vi "Control FM sweep.vi"() -> ()   [LabVIEW 2009]
doc: "A wrapper around <B>Set FM sweep.vi</B> that allows you to use either start/stop or center/span frequency controls to set up an FM sweep."
uses:
  FG FM sweep center span control.ctl
  FG FM sweep start stop control.ctl
  Magnet/Oxford/PSSUBS.LLB/PSIO.ctl
  Magnet/Oxford/BUSGEN.LLB/OxfordAddress.ctl
  Tektronix AFG 3000 Series/controls.llb/Voltage.ctl
  Tektronix AFG 3000 Series/Tektronix AFG 3000 Series.lvlib
panel:
  out "Max Delta F":dbl[unit] format="%.3g"
  in  "Overall rep rate":dbl[unit]=50.0 min=0.0 step=0.01 format="%.3g"
  in  "# frequencies":u32=3 min=1 step=1
  in  "center/span":T1 {"span" min=0.0 step=10000.0 format="%.4g"; "center" min=0.0 step=10000.0 format="%.4g"}
  in  "track B field":bool
  in  "RF on/off (ch. 1)":bool
  in  "peak-to-peak voltage":dbl[unit]=1.0 format="%.2g"
  in  "set":bool
  in  "exit":bool
  in  "start/stop":T2 {"stop" min=0.0 step=10000.0 format="%.4g"; "start" min=0.0 step=10000.0 format="%.4g"}
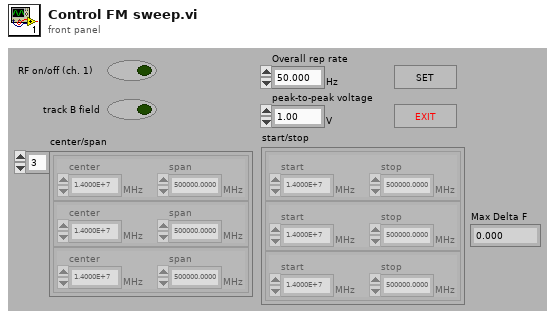
[diagram p1: front panel]
types:
  T1 = typedef "FG FM sweep center span control.ctl" = cluster{"center":dbl[unit], "span":dbl[unit]}[]
  T2 = typedef "FG FM sweep start stop control.ctl" = cluster{"start":dbl[unit], "stop":dbl[unit]}[]
  T3 = typedef "PSIO.ctl" = cluster{"Address":T4, "Version":enum16{"PS", "IPS"}}
  T4 = typedef "OxfordAddress.ctl" = cluster{"Com Port":i32, "ISOBUS Address":i32, "GPIB Address":i16, "Communication":enum16{"RS232", "ISOBUS", "GPIB", "Gateway"}}
  T5 = typedef "Voltage.ctl" = enum16{"amplitude", "offset", "high", "low", "high limit", "low limit"}
  T6 = typedef "LVRectTypeDef.ctl" = cluster{"left":i16, "top":i16, "right":i16, "bottom":i16}
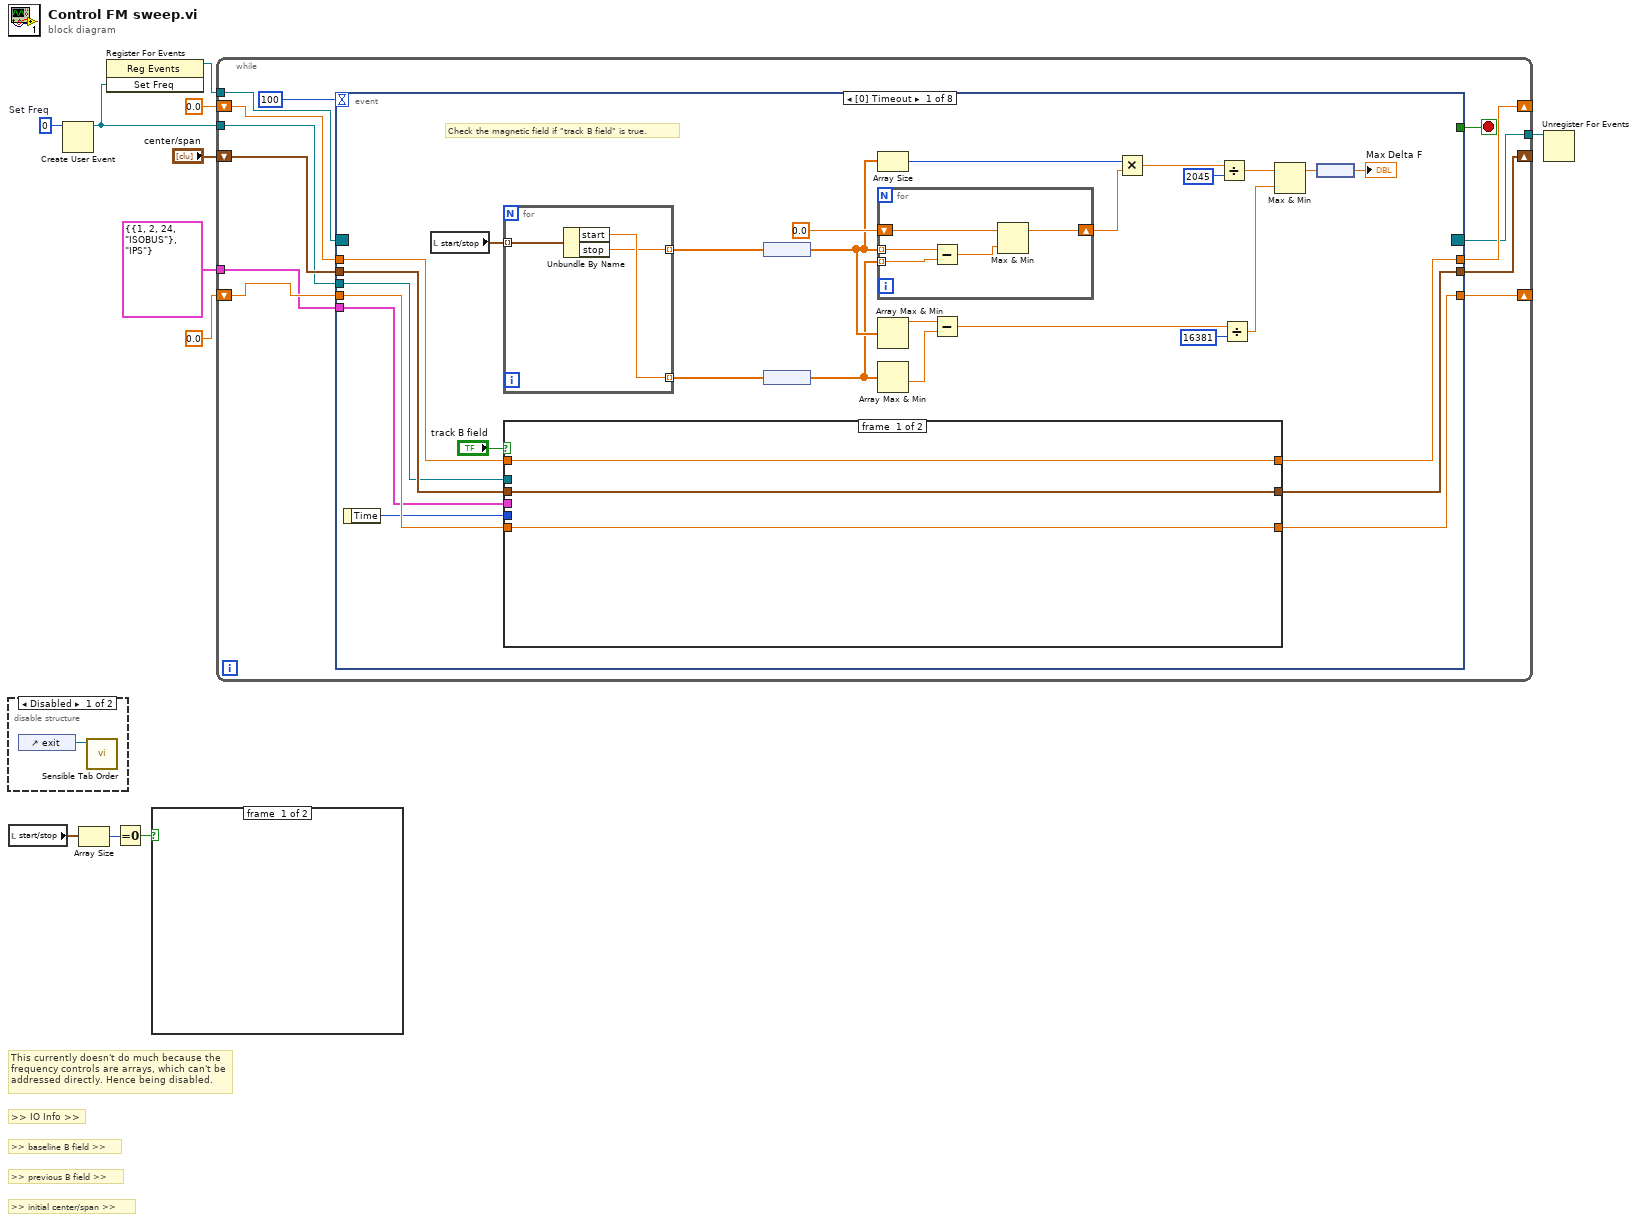
[diagram p0: block diagram]
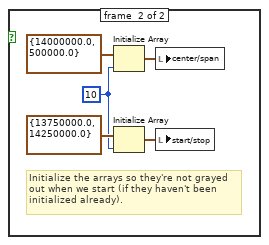
[diagram p2: hidden frame]
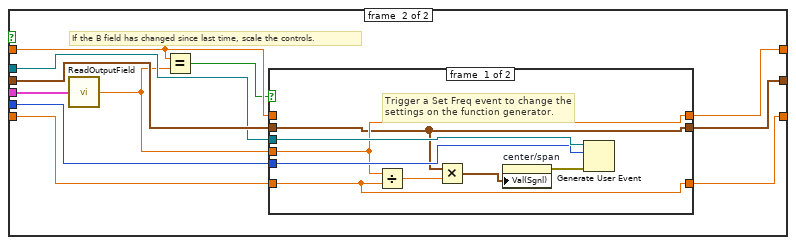
[diagram p4: hidden frame]
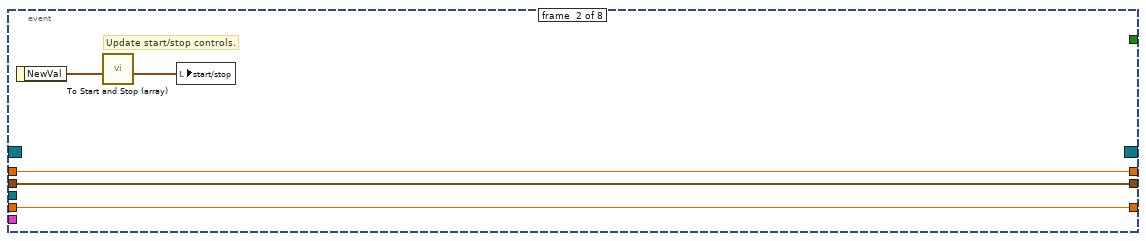
[diagram p6: hidden frame]
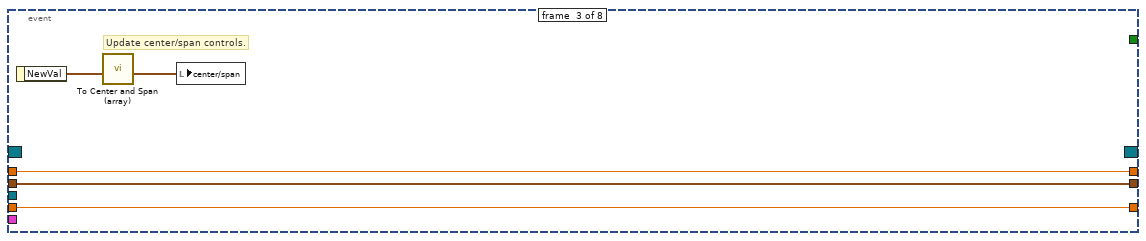
[diagram p7: hidden frame]
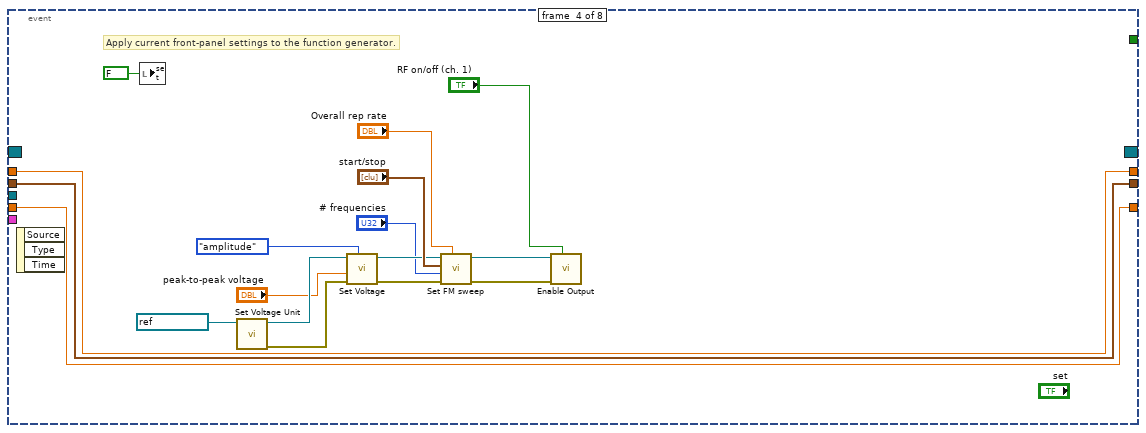
[diagram p8: hidden frame]
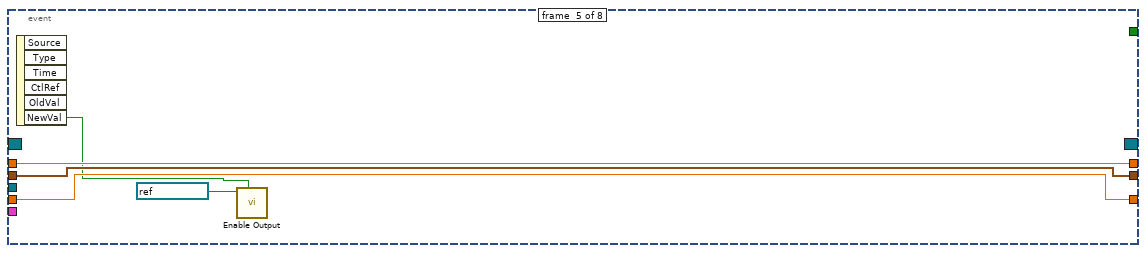
[diagram p9: hidden frame]
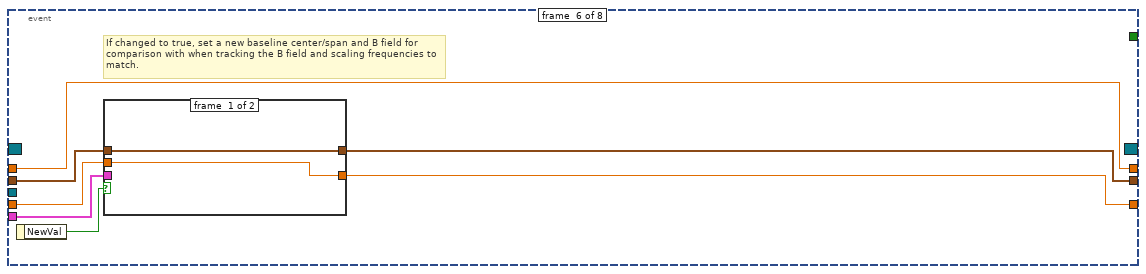
[diagram p10: hidden frame]
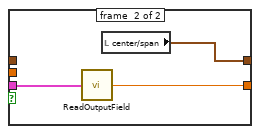
[diagram p11: hidden frame]
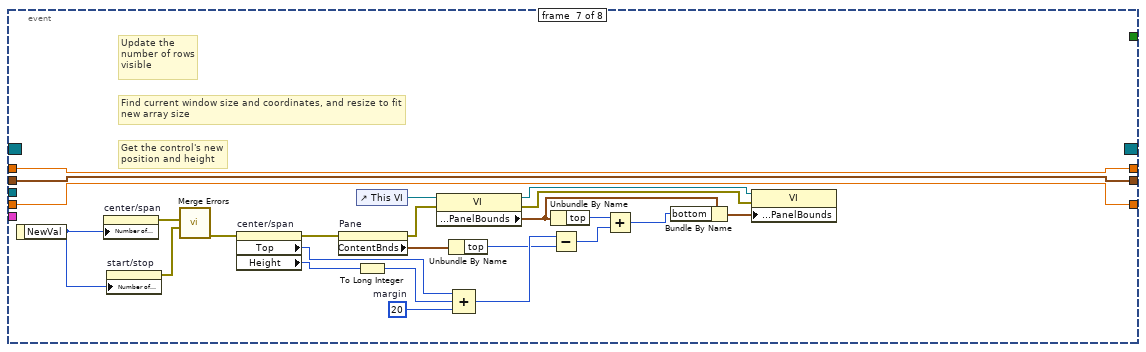
[diagram p12: hidden frame]
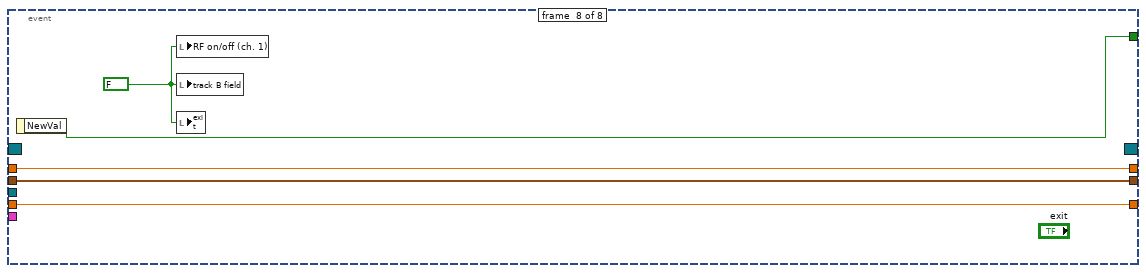
[diagram p13: hidden frame]
diagram:
  w8 = u32 0  # Set Freq
  # "This currently doesn't do much because the frequency controls are arrays, which can't be addressed directly. Hence being disabled."
  # ">> IO Info >>"
  # ">> baseline B field >>"
  # ">> previous B field >>"
  # ">> initial center/span >>"
  n1 = disable-structure shown="Disabled" {
    frame #0 {
      n2 = control-ref of="exit"() -> (w12:refnum<vi>)
      n3 = call "Sensible Tab Order.vi"("Bool Refnum"=w12) -> ()  [unwired: 11 out]
    }
    frame #1 {
    }
  }
  n4 = local read "start/stop"() -> (w5:T2)
  n5 = Create User Event(user event datatype=w8) -> (user event=w9:refnum<user-event>)  [unwired: 1 in, 1 out]
  n6 = Array Size(array=w5) -> (size(s)=w4:i32)
  n7 = register-events(w9) -> (reference out=w10:refnum<event-registration>)  [unwired: 2 in, 1 out]
  n8 = Equal To 0?(x=w4) -> (x = 0?=w3:bool)
  n9 = case shown="True" w3 {
    frame #0 {
    }
    frame #1 {
      w13 = 10 ("dimension size")
      # "Initialize the arrays so they're not grayed out when we start (if they haven't been initialized already)."
      n10 = Initialize Array(cluster{"start":dbl[unit], "stop":dbl[unit]} {"start"=14000000.0, "stop"=500000.0} ("Frequency 1"), w13) -> (w15:cluster{"start":dbl[unit], "stop":dbl[unit]}[])
      n11 = Initialize Array(cluster{"start":dbl[unit], "stop":dbl[unit]} {"start"=13750000.0, "stop"=14250000.0} ("Frequency 1"), w13) -> (w17:cluster{"start":dbl[unit], "stop":dbl[unit]}[])
      n12 = local write "center/span"(w15) -> ()
      n13 = local write "start/stop"(w17) -> ()
    }
  }
  n14 = while {
    shift-right: [w27] -> _
    shift-left: dbl[unit] 0.0 ("Field") -> [w26]
    shift-right: [w25] -> _
    shift-left: "center/span" -> [w24]
    tunnel: T3 {"Address"={"Com Port"=1, "ISOBUS Address"=2, "GPIB Address"=24, "Communication"=enum."ISOBUS"}, "Version"=enum."IPS"} ("IO Info") -> [w23]
    tunnel: w10 -> [w22]
    tunnel: w9 -> [w21]
    shift-right: [w20] -> _
    shift-left: dbl[unit] 0.0 ("last B field") -> [w19]
    tunnel: [w18] -> w6
    stop <- w29 stop-if-true
    n15 = event shown="[0] Timeout" {
      selector: w22 -> [_ _ _ _ _ _ _ _]
      dyn-events: [_ _ _ _ _ _ _ _] -> w18
      timeout: 100 -> [_ _ _ _ _ _ _ _]
      tunnel: [_ _ _ _ _ _ _ w163] -> w29
      tunnel: [w55 w95 w100 w105 w122 w126 w135 w162] -> w27
      tunnel: w26 -> [w56 w95 w100 w105 w122 w128 w135 w162]
      tunnel: [w53 w94 w99 w104 w121 w127 w136 w161] -> w25
      tunnel: w24 -> [w54 w94 w99 w104 w121 w125 w136 w161]
      tunnel: w23 -> [w52 _ _ _ _ w124 _ _]
      tunnel: w21 -> [w51 _ _ _ _ _ _ _]
      tunnel: [w49 w93 w98 w103 w120 w123 w137 w160] -> w20
      tunnel: w19 -> [w48 w93 w98 w103 w120 w123 w137 w160]
      event #0 {
        # "Check the magnetic field if \"track B field\" is true."
        n16 = event-data() -> ("Time"=w50:u32)  [unwired: 1 out]
        n17 = local read "start/stop"() -> (w47:T2)
        n18 = for {
          tunnel: w47 -> [w65] mode=indexing
          tunnel: [w64] -> w32 mode=indexing
          tunnel: [w63] -> w35 mode=indexing
          n19 = Unbundle By Name(w65) -> ("start"=w64:dbl[unit], "stop"=w63:dbl[unit])
        }
        n20 = case shown="True" "track B field" {
          tunnel: w56 -> [w68 w79]
          tunnel: [w68 w70] -> w55
          tunnel: w54 -> [w67 w78]
          tunnel: [w67 w69] -> w53
          tunnel: w52 -> [_ w77]
          tunnel: w51 -> [_ w76]
          tunnel: w50 -> [_ w75]
          tunnel: [w66 w73] -> w49
          tunnel: w48 -> [w66 w72]
          frame #0 {
          }
          frame #1 {
            # "If the B field has changed since last time, scale the controls."
            n21 = call "ReadOutputField.vi"("IO Info"=w77) -> ("Field"=w74:dbl[unit])  [unwired: 2 out]
            n22 = Equal?(x=w72, y=w74) -> (x = y?=w71:bool)
            n23 = case shown="False" w71 {
              tunnel: w79 -> [w81 w89]
              tunnel: w78 -> [w80 w88]
              tunnel: w76 -> [w85 _]
              tunnel: w75 -> [w84 _]
              tunnel: w74 -> [w82 _]
              tunnel: [w82 w90] -> w73
              tunnel: w72 -> [_ w90]
              tunnel: [w81 w89] -> w70
              tunnel: [w80 w88] -> w69
              frame #0 {
                # "Trigger a Set Freq event to change the settings on the function generator."
                n24 = Divide(x=w82, y=w81) -> (x/y=w87:dbl)
                n25 = Multiply(x=w80, y=w87) -> (x*y=w86:T1)
                n26 = property on="center/span" class="Arr (strict)"("Val(Sgnl)"=w86) -> (error out=w83:errorcluster)  [unwired: 2 in, 1 out]
                n27 = Generate User Event(user event=w85, event data cluster=w84, error in=w83) -> ()  [unwired: 2 out]
              }
              frame #1 {
              }
            }
          }
        }
        n28 = node(w35) -> (w34:dbl[])
        n29 = node(w32) -> (w33:dbl[])
        n30 = Array Size(array=w34) -> (size(s)=w46:i32)
        n31 = for {
          tunnel: w34 -> [w62] mode=indexing
          tunnel: w33 -> [w61] mode=indexing
          shift-right: [w59] -> w36
          shift-left: 0.0 -> [w58]
          n32 = Subtract(x=w62, y=w61) -> (x-y=w60:dbl)
          n33 = Max & Min(x=w58, y=w60) -> (max(x,y)=w59:dbl)  [unwired: 1 out]
        }
        n34 = Array Max & Min(array=w34) -> (max value=w40:dbl)  [unwired: 3 out]
        n35 = Array Max & Min(array=w33) -> (min value=w41:dbl)  [unwired: 3 out]
        n36 = Subtract(x=w40, y=w41) -> (x-y=w42:dbl)
        n37 = Multiply(x=w46, y=w36) -> (x*y=w38:dbl)
        n38 = Divide(x=w38, y=2045) -> (x/y=w44:dbl)
        n39 = Divide(x=w42, y=16381) -> (x/y=w45:dbl)
        n40 = Max & Min(x=w44, y=w45) -> (max(x,y)=w31:dbl)  [unwired: 1 out]
        n41 = node(w31) -> (→"Max Delta F":dbl[unit])
      }
      event #1 {
        # "Update start/stop controls."
        n42 = event-data() -> ("NewVal"=w92:T1)  [unwired: 1 out]
        n43 = call "To Start and Stop (array).vi"("center/span"=w92) -> ("start/stop"=w91:T2)  [unwired: 6 out]
        n44 = local write "start/stop"(w91) -> ()
      }
      event #2 {
        # "Update center/span controls."
        n45 = event-data() -> ("NewVal"=w97:T2)  [unwired: 1 out]
        n46 = call "To Center and Span (array).vi"("start/stop"=w97) -> ("center/span"=w96:T1)  [unwired: 6 out]
        n47 = local write "center/span"(w96) -> ()
      }
      event #3 {
        # "Apply current front-panel settings to the function generator."
        n48 = event-data() -> ()  [unwired: 4 out]
        n49 = local write "set"(FALSE) -> ()
        n50 = call "Set Voltage Unit.vi"("VISA resource name"=refnum<visa-resource-name> "AFG3252") -> ("error out"=w113:errorcluster, "VISA resource name out"=w114:refnum<visa-resource-name>)  [unwired: 3 in, 6 out]
        n51 = call "Set Voltage.vi"("Voltage Param (amplitude)"=Voltage."amplitude", "error in (no error)"=w113, "voltage"="peak-to-peak voltage", "VISA resource name"=w114) -> ("error out"=w109:errorcluster, "VISA resource name out"=w110:refnum<visa-resource-name>)  [unwired: 1 in, 5 out]
        n52 = call "Set FM sweep.vi"("Overall rep rate"="Overall rep rate", "error in (no error)"=w109, "# frequencies"="# frequencies", "Start/stop frequencies"="start/stop", "VISA resource name"=w110) -> ("error out"=w106:errorcluster, "VISA resource name out"=w107:refnum<visa-resource-name>)  [unwired: 5 out]
        n53 = call "Enable Output.vi"("Enable Output (T: Enable)"="RF on/off (ch. 1)", "error in (no error)"=w106, "VISA resource name"=w107) -> ()  [unwired: 1 in, 8 out]
      }
      event #4 {
        n54 = event-data() -> ("NewVal"=w119:bool)  [unwired: 6 out]
        n55 = call "Enable Output.vi"("Enable Output (T: Enable)"=w119, "VISA resource name"=refnum<visa-resource-name> "AFG3252") -> ()  [unwired: 2 in, 8 out]
      }
      event #5 {
        # "If changed to true, set a new baseline center/span and B field for comparison with when tracking the B field and scaling frequencies to match."
        n56 = event-data() -> ("NewVal"=w129:bool)  [unwired: 1 out]
        n57 = case shown="False" w129 {
          tunnel: w128 -> [w131 _]
          tunnel: [w130 w134] -> w127
          tunnel: [w131 w132] -> w126
          tunnel: w125 -> [w130 _]
          tunnel: w124 -> [_ w133]
          frame #0 {
          }
          frame #1 {
            n58 = call "ReadOutputField.vi"("IO Info"=w133) -> ("Field"=w132:dbl[unit])  [unwired: 2 out]
            n59 = local read "center/span"() -> (w134:T1)
          }
        }
      }
      event #6 {
        w146 = 20  # margin
        # "Find current window size and coordinates, and resize to fit new array size"
        # "Get the control's new position and height"
        # "Update the number of rows visible"
        n60 = event-data() -> ("NewVal"=w138:u32)  [unwired: 1 out]
        n61 = property on="center/span" class="Arr (strict)"("Number of Rows"=w138) -> (error out=w158:errorcluster)  [unwired: 2 in, 1 out]
        n62 = property on="start/stop" class="Arr (strict)"("Number of Rows"=w138) -> (error out=w157:errorcluster)  [unwired: 2 in, 1 out]
        n63 = call <vilib>:"Merge Errors.vi"("error in 3 (no error)"=w157, "error in 2 (no error)"=w158) -> ("error out"=w152:errorcluster)  [unwired: 2 in, 3 out]
        n64 = property on="center/span" class="Arr (strict)"(error in=w152) -> (error out=w154:errorcluster, "Top"=w155:i32, "Height"=w153:u32)  [unwired: 1 in, 1 out]
        n65 = property on="Pane" class="Pane"(error in=w154) -> (error out=w156:errorcluster, "ContentBnds"=w151:T6)  [unwired: 1 in, 1 out]
        n66 = control-ref of="This VI"() -> (w149:refnum<vi>)
        n67 = To Long Integer(number=w153) -> (32bit integer=w150:i32)
        n68 = property class="VI"(reference=w149, error in=w156) -> (reference out=w148:refnum<vi>, error out=w139:errorcluster, "Front Panel.PanelBounds"=w143:T6)
        n69 = Unbundle By Name(w151) -> ("top"=w144:i16)
        n70 = Compound Arithmetic op=ADD(w155, w150, w146) -> (w145:i32)
        n71 = Unbundle By Name(w143) -> ("top"=w142:i16)
        n72 = Subtract(x=w145, y=w144) -> (x-y=w141:i32)
        n73 = Add(x=w142, y=w141) -> (x+y=w140:i32)
        n74 = Bundle By Name(cluster=w143, "bottom"=w140) -> (w147:T6)
        n75 = property class="VI"(reference=w148, error in=w139, "Front Panel.PanelBounds"=w147) -> ()  [unwired: 2 out]
      }
      event #7 {
        w159 = FALSE
        n76 = event-data() -> ("NewVal"=w163:bool)  [unwired: 1 out]
        n77 = local write "RF on/off (ch. 1)"(w159) -> ()
        n78 = local write "track B field"(w159) -> ()
        n79 = local write "exit"(w159) -> ()
      }
    }
  }
  n80 = Unregister For Events(event registration refnum=w6) -> ()  [unwired: 1 in, 1 out]
